vi "auto datalogger user selected.vi"(9 "data log interval (s)":sgl=1.0 min=1, 11 "datalog ref":refnum<file>) -> (0 "File Failure":bool, 3 "File refnum":refnum<file>)   [LabVIEW 2015]
uses:
  DAQ configuration/Sensor buffer command.ctl
  logic buffer cmd.ctl
  calibration/Shared Data/buffer.ctl
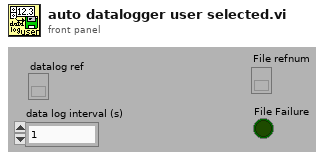
[diagram p1: front panel]
types:
  T1 = typedef "buffer.ctl" = enum16{"write", "read", "read merge"}
  T2 = typedef "logic buffer cmd.ctl" = enum16{"read", "write ouput settings", "write rules", "write setpoints", "write output descriptions", "write all", "calculate setpoints", "save", "open", "Load all setpoint code", "Load one setpoint code", "Configure one setpoint code"}
  T3 = typedef "Sensor buffer command.ctl" = enum16{"read average", "read recent", "read all", "write", "set buffer size", "Read channel config", "Write channel config", "clear"}
  T4 = typedef "Sensor data.ctl" = cluster{" Sensor array":T5[], "Time":dbl}
  T5 = typedef "sensor cluster.ctl" = cluster{"voltage":sgl, "scaled":sgl, "units":string, "Out of Range":bool}
  T6 = typedef "variable setpoint.ctl" = cluster{"name":string, "unit":string, "value":dbl, "Type":enum16{"Constant", "Variable"}, "variable":cluster{"selected sensors":i32[], "selected set points":i32[], "VI":path, "Data average interval":T7, "code ref":T8}}
  T7 = typedef "data ave interval.ctl" = dbl
  T8 = typedef "type specifier for control code.ctl" = refnum<vi>
  T9 = typedef "Channel config.ctl" = cluster{"Channel Indices":T10[], "AI Max voltage":dbl[], "Calibration matrix":T11}
  T10 = typedef "channel identifier.ctl" = u16
  T11 = typedef "calib array.ctl" = T12[]
  T12 = typedef "conversion.ctl" = cluster{"conversion matrix":sgl[][], "units":string, "name":string, "scale type":T13, "offset (volts)":dbl, "second channel":i8, "correspondence table":T14, "offset (physical units)":dbl, "pH scale":T15, "D.O.":T16, "Photometer data":T17}
  T13 = typedef "scale type.ctl" = enum16{"Volts", "Polynomial", "Correspondence Table", "pH", "Dissolved Oxygen", "Quadratic", "Photometer"}
  T14 = typedef "correspondence table.ctl" = cluster{"physical units":dbl, "volts":dbl}[]
  T15 = typedef "pH scale.ctl" = cluster{"Buffers":cluster{"Buffer":dbl, "Calibrated":bool, "V/T":dbl}[], "Temperature":dbl}
  T16 = typedef "DO scale.ctl" = cluster{"Temperature":dbl, "K":dbl, "barometric pressure":dbl}
  T17 = typedef "Photometer calibration data.ctl" = cluster{"Dark Voltage":dbl, "Blank Voltage":dbl, "Standards":cluster{"Concentration":dbl, "Voltage":dbl}[]}
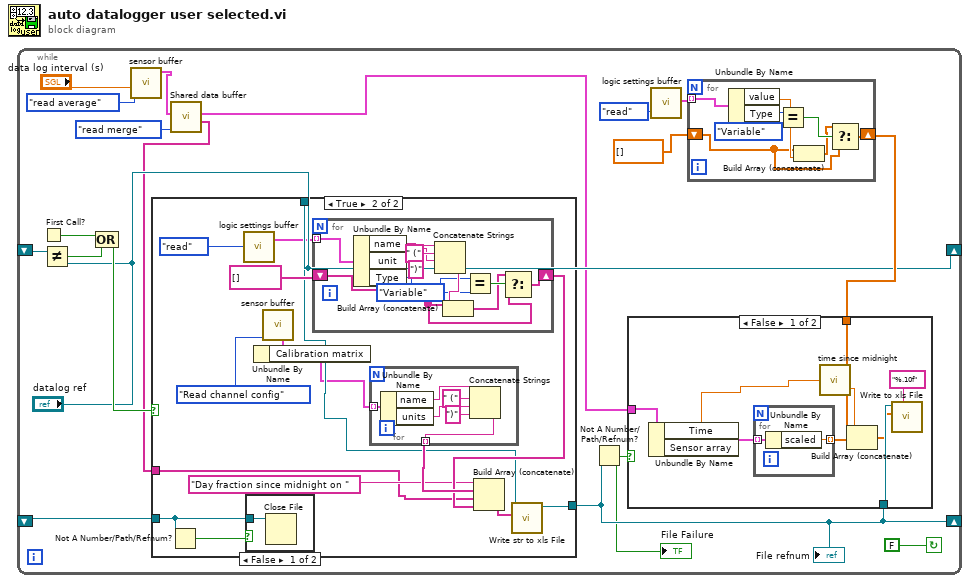
[diagram p0: block diagram]
diagram:
  n1 = while {
    shift-left: _ -> [w19]
    shift-right: ["datalog ref"] -> _
    shift-right: [w15] -> _
    shift-left: _ -> [w14]
    stop <- FALSE continue-if-true
    n2 = First Call?() -> (First Call?: T/F=w17:bool)
    n3 = Not Equal?(x=w19, y="datalog ref") -> (x != y?=w16:bool)
    n4 = Compound Arithmetic op=OR(w17, w16) -> (w13:bool)
    n5 = call "sensor buffer.vi"("command"=Sensor_buffer_command."read average", "smooth interval (s)"="data log interval (s)") -> ("Calibrated data"=w3:T4)  [unwired: 5 in, 4 out]
    n6 = call "Shared data buffer.vi"("command"=buffer."read merge", "Data from local sources in"=w3) -> ("Shared data names (unit) out"=w1:string[], "Data from merged sources out"=w2:T4)  [unwired: 7 in, 1 out]
    n7 = case shown="True" w13 {
      tunnel: w14 -> [w28 w41]
      tunnel: [w28 w43] -> w15
      tunnel: "datalog ref" -> [_ w36]
      tunnel: w1 -> [_ w29]
      frame False {
      }
      frame True {
        n8 = Not A Number/Path/Refnum?(number/path/refnum=w41) -> (NaN/Path/Refnum?=w40:bool)
        n9 = call "logic settings buffer.vi"("command"=logic_buffer_cmd."read") -> ("Set Points out"=w33:T6[])  [unwired: 11 in, 7 out]
        n10 = case shown="False" w40 {
          tunnel: w41 -> [w56 _]
          frame False {
            n11 = Close File(refnum=w56) -> ()  [unwired: 1 in, 2 out]
          }
          frame True {
          }
        }
        n12 = call "sensor buffer.vi"("command"=Sensor_buffer_command."Read channel config") -> ("Channel Config out"=w32:T9)  [unwired: 6 in, 4 out]
        n13 = Unbundle By Name(w32) -> ("Calibration matrix"=w30:T11)
        n14 = for {
          tunnel: w33 -> [w55] mode=indexing
          shift-right: [w44] -> w37
          shift-left: string[] [] -> [w45]
          n15 = Unbundle By Name(w55) -> ("name"=w52:string, "unit"=w51:string, "Type"=w48:enum16{"Constant", "Variable"})
          n16 = Concatenate Strings(w52, " (" ("Substring"), w51, ")" ("Substring")) -> (w49:string)
          n17 = Build Array (concatenate)(w45, w49) -> (w46:string[])
          n18 = Equal?(x=w48, y=enum16{"Constant", "Variable"}."Variable") -> (x = y?=w50:bool)
          n19 = Select(t=w46, s=w50, f=w45) -> (s? t:f=w44:string[])
        }
        n20 = for {
          tunnel: w30 -> [w62] mode=indexing
          tunnel: [w57] -> w42 mode=indexing
          n21 = Unbundle By Name(w62) -> ("name"=w61:string, "units"=w59:string)
          n22 = Concatenate Strings(w61, " (" ("Substring"), w59, ")" ("Substring")) -> (w57:string)
        }
        n23 = Build Array (concatenate)("Day fraction since midnight on " ("Substring"), w42, w29, w37) -> (w34:string[])
        n24 = call "Write str to xls File.vi"("1D data"=w34, "refnum"=w36) -> ("dup refnum"=w43:refnum<file>)  [unwired: 8 in, 1 out]
      }
    }
    "File refnum" <- w15
    n25 = Not A Number/Path/Refnum?(number/path/refnum=w15) -> (NaN/Path/Refnum?=w12:bool)
    "File Failure" <- w12
    n26 = call "logic settings buffer.vi"("command"=logic_buffer_cmd."read") -> ("Set Points out"=w8:T6[])  [unwired: 11 in, 7 out]
    n27 = for {
      tunnel: w8 -> [w27] mode=indexing
      shift-right: [w21] -> w6
      shift-left: dbl[] [] -> [w20]
      n28 = Unbundle By Name(w27) -> ("value"=w23:dbl, "Type"=w26:enum16{"Constant", "Variable"})
      n29 = Equal?(x=w26, y=enum16{"Constant", "Variable"}."Variable") -> (x = y?=w24:bool)
      n30 = Build Array (concatenate)(w20, w23) -> (w22:dbl[])
      n31 = Select(t=w22, s=w24, f=w20) -> (s? t:f=w21:dbl[])
    }
    n32 = case shown="False" w12 {
      tunnel: w15 -> [w68 _]
      tunnel: w2 -> [w65 _]
      tunnel: w6 -> [w64 _]
      frame False {
        n33 = Unbundle By Name(w65) -> ("Time"=w67:dbl, "Sensor array"=w70:T5[])
        n34 = for {
          tunnel: w70 -> [w73] mode=indexing
          tunnel: [w72] -> w69 mode=indexing
          n35 = Unbundle By Name(w73) -> ("scaled"=w72:sgl)
        }
        n36 = call "time since midnight.vi"("seconds since 1Jan1904"=w67) -> ("Days"=w66:dbl)  [unwired: 1 out]
        n37 = Build Array (concatenate)(w66, w69, w64) -> (w63:dbl[])
        n38 = call "Write to xls File.vi"("format (%.3f)"="%.10f", "1D data"=w63, "refnum"=w68) -> ()  [unwired: 7 in, 2 out]
      }
      frame True {
      }
    }
  }
